vi "positionManager.vi"(5 "Display":i32=1, 6 "Reverse Y":bool=TRUE, 7 "Reverse X":bool, 9 "Cluster":T1={"Xoffset"=100.0, "Yoffset in"=0.0, "X position in"=-2.9872204472843453, "Y position in"=0.9349593495934956, "Fine X position"=-0.8785942492012779, "Fine Y position"=2.6518218623481786} {"Fine Y position" scale=0.0..10.0; "Fine X position" scale=0.0..10.0; "Y position in" scale=0.0..10.0; "X position in" scale=0.0..10.0}) -> (0 "Y position out":dbl=60.00707679141567, 1 "X position out":dbl=-53.75399361022366, 3 "output cluster":cluster{i32, i32}={-54, 60})   [LabVIEW 2022 SP3]
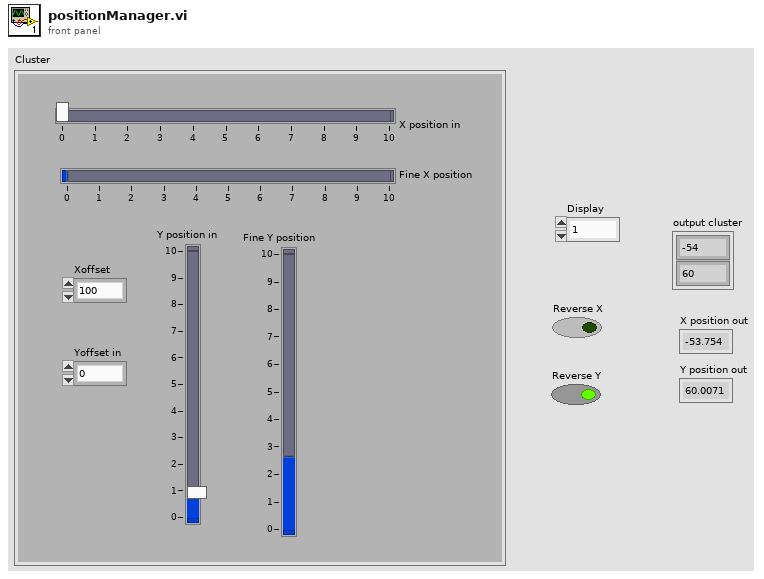
[diagram p1: front panel]
types:
  T1 = cluster{"Xoffset":dbl, "Yoffset in":dbl, "X position in":dbl, "Y position in":dbl, "Fine X position":dbl, "Fine Y position":dbl}
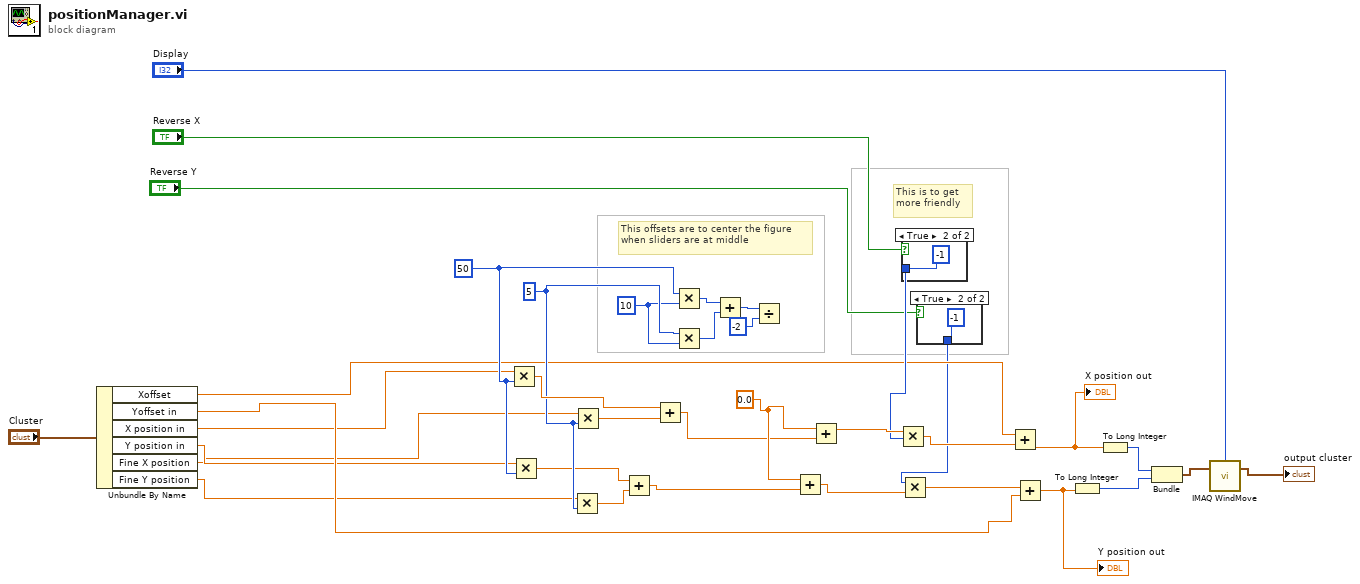
[diagram p0: block diagram]
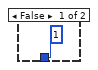
[diagram p2: hidden frame]
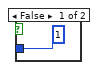
[diagram p3: hidden frame]
diagram:
  w36 = 0.0 ("x")
  w19 = 10 ("y")
  w20 = 5
  w18 = 50
  # "This is to get more friendly"
  # "This offsets are to center the figure when sliders are at middle"
  n1 = Unbundle By Name("Cluster") -> ("Xoffset"=w13:dbl, "Yoffset in"=w12:dbl, "X position in"=w11:dbl, "Y position in"=w10:dbl, "Fine X position"=w9:dbl, "Fine Y position"=w8:dbl)
  n2 = Multiply(x=w11, y=w18) -> (x*y=w25:dbl)
  n3 = Multiply(x=w10, y=w18) -> (x*y=w16:dbl)
  n4 = Multiply(x=w8, y=w20) -> (x*y=w17:dbl)
  n5 = Multiply(x=w9, y=w20) -> (x*y=w26:dbl)
  n6 = Add(x=w16, y=w17) -> (x+y=w28:dbl)
  n7 = Add(x=w25, y=w26) -> (x+y=w27:dbl)
  n8 = Multiply(x=w18, y=w19) -> (x*y=w21:i32)
  n9 = Multiply(x=w20, y=w19) -> (x*y=w22:i32)
  n10 = Add(x=w21, y=w22) -> (x+y=w23:i32)
  n11 = Divide(x=w23, y=-2) -> ()  [unwired: 1 out]
  n12 = Add(x=w36, y=w28) -> (x+y=w31:dbl)
  n13 = Add(x=w36, y=w27) -> (x+y=w30:dbl)
  n14 = case shown="True" "Reverse X" {
    tunnel: [1 ("y") -1 ("y")] -> w29
    frame False {
    }
    frame True {
    }
  }
  n15 = Multiply(x=w30, y=w29) -> (x*y=w32:dbl)
  n16 = case shown="True" "Reverse Y" {
    tunnel: [1 ("y") -1 ("y")] -> w1
    frame False {
    }
    frame True {
    }
  }
  n17 = Multiply(x=w1, y=w31) -> (x*y=w33:dbl)
  n18 = Add(x=w13, y=w32) -> (x+y=w7:dbl)
  "X position out" <- w7
  n19 = Add(x=w33, y=w12) -> (x+y=w6:dbl)
  "Y position out" <- w6
  n20 = To Long Integer(number=w6) -> (32bit integer=w35:i32)
  n21 = To Long Integer(number=w7) -> (32bit integer=w34:i32)
  n22 = Bundle(w34, w35) -> (w3:cluster{i32, i32})  [unwired: 1 in]
  n23 = call "IMAQ WindMove"("Window Number (0...15)"="Display", "Coordinates (screen)"=w3) -> ("Coordinates (screen)"=→"output cluster":cluster{"X Position":i32, "Y Position":i32})  [unwired: 3 in, 1 out]
